vi "Test1.vi"() -> ()   [LabVIEW 2011]
panel:
  in  "address":string="192.168.254.112"
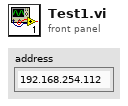
[diagram p1: front panel]
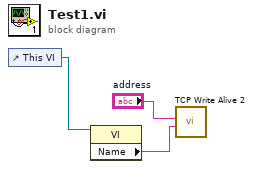
[diagram p0: block diagram]
diagram:
  n1 = control-ref of="This VI"() -> (w3:refnum<vi>)
  n2 = property class="VI"(reference=w3) -> ("Name"=w2:string)  [unwired: 1 in, 2 out]
  n3 = call "TCP Write Alive 2.vi"("Name"=w2, "address"="address") -> ()  [unwired: 10 in]
